vi "Analysis.Result Summaries, Generate Yield Per Day_V2a.vi"(10 "Yield":dbl[](array[numeric]), 11 "Dates":timestamp[](array[timestamp])) -> (2 "Yield Per Date":string[][](table), 3 "Yield vs Date":cluster{"Dates":timestamp[], "Yield":dbl[]}(graph))   [LabVIEW 2024]
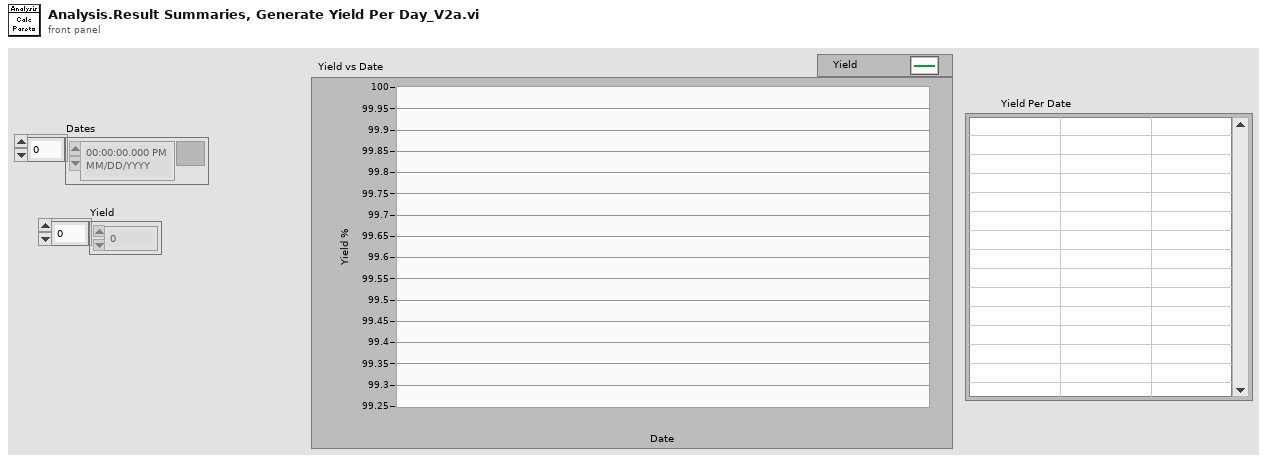
[diagram p1: front panel]
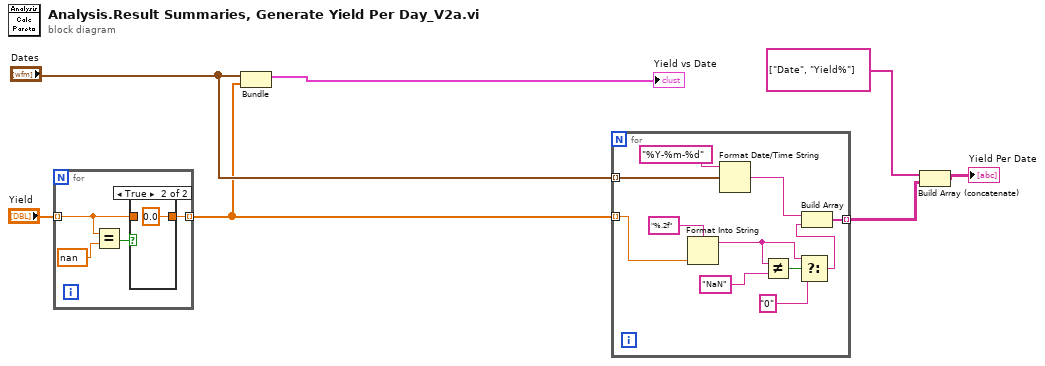
[diagram p0: block diagram]
diagram:
  n1 = for {
    tunnel: "Yield" -> [w9] mode=indexing
    tunnel: [w8] -> w1 mode=indexing
    n2 = Equal?(x=w9, y=nan) -> (x = y?=w10:bool)
    n3 = case shown="True" w10 {
      tunnel: w9 -> [w12 _]
      tunnel: [w12 0.0 ("Numeric")] -> w8
      frame False {
      }
      frame True {
      }
    }
  }
  n4 = Bundle("Dates"="Dates", w1) -> (→"Yield vs Date":cluster{"Dates":timestamp[], dbl[]})  [unwired: 1 in]
  n5 = for {
    tunnel: w1 -> [w22] mode=indexing
    tunnel: "Dates" -> [w24] mode=indexing
    tunnel: [w19] -> w7 mode=indexing
    n6 = Format Into String(format string="%.2f", w22) -> (resulting string=w16:string)  [unwired: 2 in, 1 out]
    n7 = Format Date/Time String(time format string (%c)="%Y-%m-%d", seconds (now)=w24) -> (date/time string=w20:string)  [unwired: 1 in]
    n8 = Not Equal?(x=w16, y="NaN") -> (x != y?=w17:bool)
    n9 = Select(t=w16, s=w17, f="0") -> (s? t:f=w15:string)
    n10 = Build Array(w20, w15) -> (w19:string[])
  }
  n11 = Build Array (concatenate)(string[] ["Date", "Yield%"], w7) -> (→"Yield Per Date":string[][])
